vi "ge_FindFPCtrl.vi"(4 "Ctrl Name":string, 5 "FP Ctrl":T1) -> (2 "Ctrl Ref":refnum<vi>)   [LabVIEW 2018]
uses:
  Custom Ctrls/ge_FPCtrlRefLabel.ctl
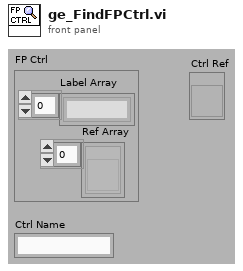
[diagram p1: front panel]
types:
  T1 = typedef "ge_FPCtrlRefLabel.ctl" = cluster{"Label Array":string[], "Ref Array":refnum<vi>[]}
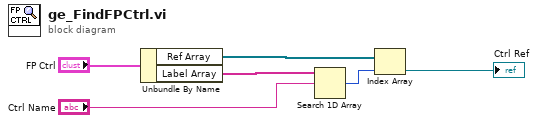
[diagram p0: block diagram]
diagram:
  n1 = Unbundle By Name("FP Ctrl") -> ("Ref Array"=w3:refnum<vi>[], "Label Array"=w4:string[])
  n2 = Search 1D Array(1D array=w4, element="Ctrl Name") -> (index of element=w2:i32)  [unwired: 1 in]
  n3 = Index Array(array=w3, index=w2) -> (element=→"Ctrl Ref":refnum<vi>)
